vi "TrackerConfig.vi"() -> ()   [LabVIEW 2011]
panel:
  out "Output":string[][](array[string])
  in  "PORT NAME":string="TrackerConfig"
  in  "Desired Address":i32=101
  in  "Current Address":i32=1
  # "Instruction"
  # "Response"
  # "Comment"
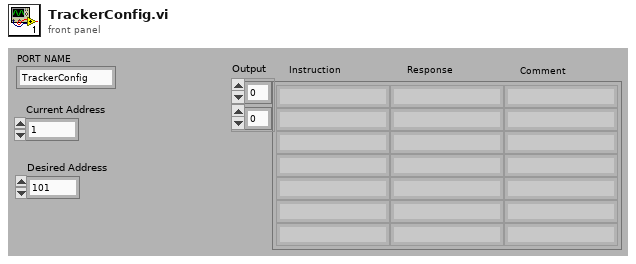
[diagram p1: front panel]
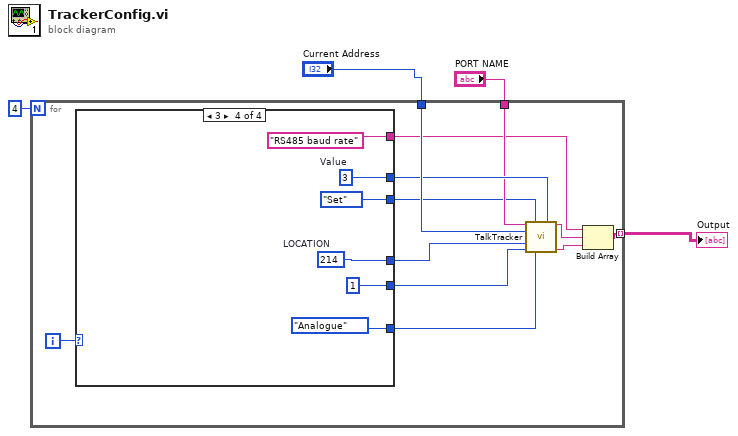
[diagram p0: block diagram]
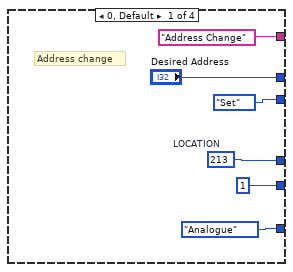
[diagram p2: hidden frame]
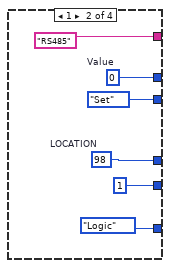
[diagram p3: hidden frame]
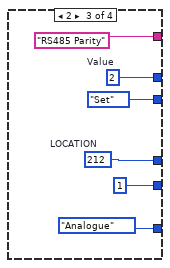
[diagram p4: hidden frame]
diagram:
  n1 = for {
    N: 4 -> [_]
    tunnel: "Current Address" -> [w15]
    tunnel: "PORT NAME" -> [w13]
    tunnel: [w8] -> w1 mode=indexing
    i -> [w16]
    n2 = case shown="3" w16 {
      tunnel: ["Desired Address" w26 w32 w38] -> w14
      tunnel: [w21 w28 w34 w40] -> w12
      tunnel: [1 ("NO. LOCATIONS") 1 ("NO. LOCATIONS") 1 ("NO. LOCATIONS") 1 ("NO. LOCATIONS")] -> w11
      tunnel: ["Address Change" "RS485" "RS485 Parity" "RS485 baud rate"] -> w9
      tunnel: [enum16{"Logic", "Analogue"}."Analogue" ("Analogue") enum16{"Logic", "Analogue"}."Logic" ("Analogue") enum16{"Logic", "Analogue"}."Analogue" ("Analogue") enum16{"Logic", "Analogue"}."Analogue" ("Analogue")] -> w7
      tunnel: [enum16{"Set", "Read"}."Set" ("Set") enum16{"Set", "Read"}."Set" ("Set") enum16{"Set", "Read"}."Set" ("Set") enum16{"Set", "Read"}."Set" ("Set")] -> w6
      frame 0, Default {
        w21 = 213  # LOCATION
        # "Address change"
      }
      frame 1 {
        w26 = 0  # Value
        w28 = 98  # LOCATION
      }
      frame 2 {
        w32 = 2  # Value
        w34 = 212  # LOCATION
      }
      frame 3 {
        w38 = 3  # Value
        w40 = 214  # LOCATION
      }
    }
    n3 = call "TalkTracker.vi"("PORT NAME"=w13, "Set"=w6, "Value to set"=w14, "MODULE ADDRESS"=w15, "LOCATION"=w12, "NO. LOCATIONS"=w11, "Analogue"=w7) -> ("Response"=w5:string, "Comment out"=w10:string)  [unwired: 6 in, 1 out]
    n4 = Build Array(w9, w5, w10) -> (w8:string[])
  }
  "Output" <- w1
